vi "MeasurementControl - Main (CLTC-C0NBTZ1's conflicted copy 2015-04-20).vi"() -> ()   [LabVIEW 2013]
uses:
  Instrument Control Switches.ctl
  Timing and Stabilization/Stabilization.ctl
  avantesSpectrometer/Acquisition/Sphere Indicator.ctl
  Time Left.ctl
  controls/Metadata all typedef.ctl
  controls/Metadata typedef.ctl
  controls/Metadata disable typedef.ctl
  CaliforniaInstrumentsIxSeries/controls/electrical2.ctl
  avantesSpectrometer/Acquisition/AvaSpec Color Parameters.ctl
  MeasurementControl Message Queue Folder/MeasurementControl Message Queue.lvlib
  avantesSpectrometer/AvaSpec.lvlib
  controls/Metadata.lvlib
  CaliforniaInstrumentsIxSeries/Acquisition/Cal Inst Acquisition.lvlib
  MR 16 teardown/MR16TestStandDAQ/Controls/Stabilization.ctl
  Timing and Stabilization.lvlib
panel:
  in  "Instrument Control Switches":T1
  in  "Exit":bool
  out "Status":string
  in  "test cal inst":bool
  in  "test Yokogawa":bool
  in  "Test Naked Sphere":bool
  in  "Start LM-79\nNaked Sphere":bool
  in  "Take Measurements\nfor Database":bool
  in  "Tab Control":T2(tab)
  out "Naked Sphere Stabilization Data":T3={"Stabilization waveform"={"t0"=timestamp(0 s since 1904-01-01), "dt"=50.0, "Y"=[10.0, 9.0, 8.75, 8.5, 8.25, 8.125, 8.06, 8.03, 8.015, 8.0, 8.0, 8.0]}, "Variation"=0.0, "Stabilized"=FALSE, "Threshold"=0.0, "time to stabilize"=0.0, "3 points"=[], "Sphere Indicator"=enum."Naked Sphere"}
  out "Insulated Sphere Stabilization Data":T3={"Stabilization waveform"={"t0"=timestamp(0 s since 1904-01-01), "dt"=50.0, "Y"=[10.0, 9.0, 8.75, 8.5, 8.25, 8.125, 8.06, 8.03, 8.015, 8.0, 8.0, 8.0]}, "Variation"=0.0, "Stabilized"=FALSE, "Threshold"=0.0, "time to stabilize"=0.0, "3 points"=[], "Sphere Indicator"=enum."Naked Sphere"}
  out "Time Left":T5
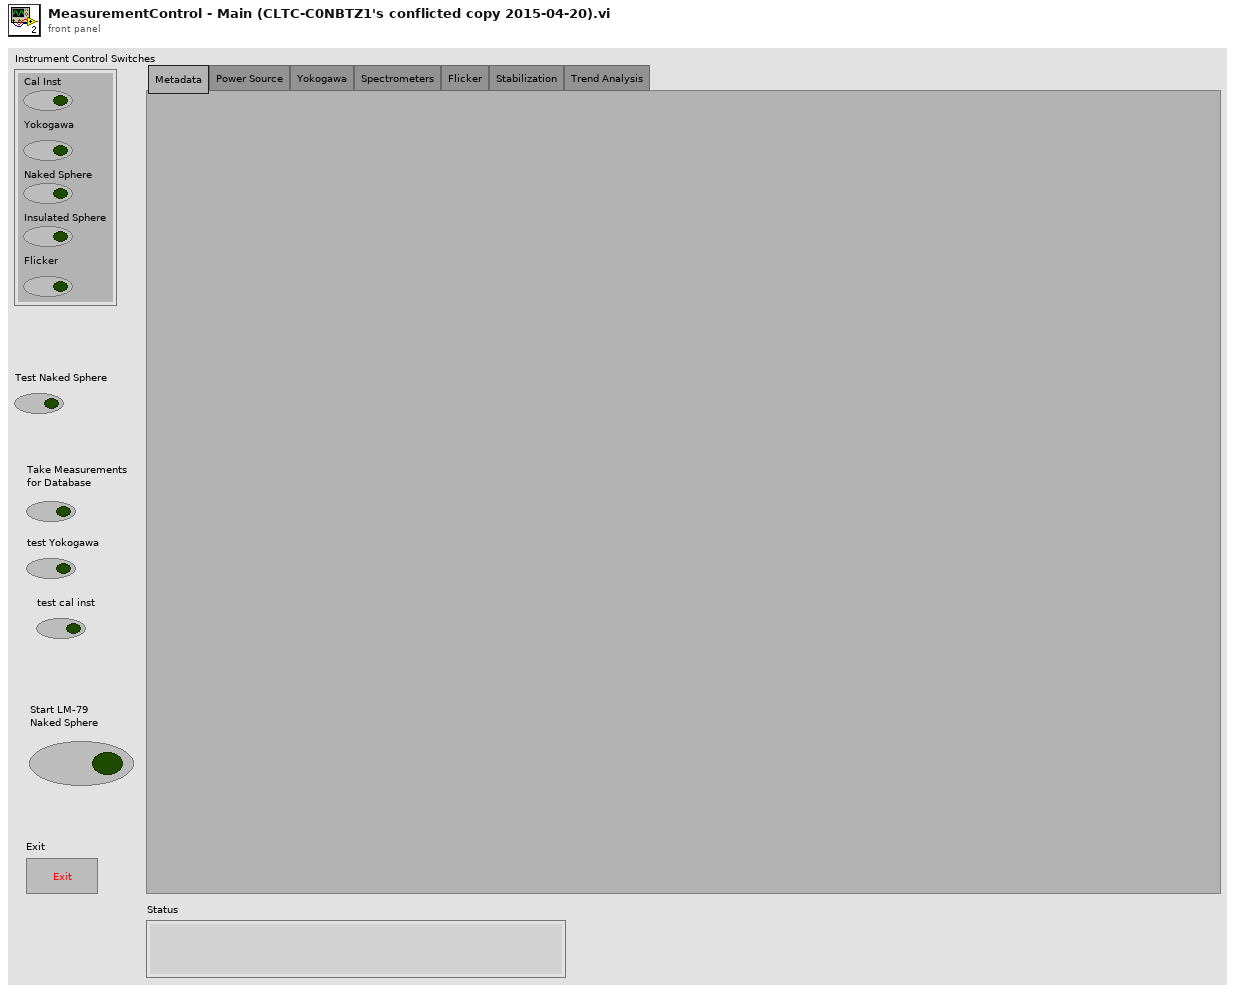
[diagram p1: front panel]
types:
  T1 = typedef "Instrument Control Switches.ctl" = cluster{"Cal Inst":bool, "Yokogawa":bool, "Naked Sphere":bool, "Insulated Sphere":bool, "Flicker":bool}
  T2 = enum32{"Metadata", "Power Source", "Yokogawa", "Spectrometers", "Flicker", "Stabilization", "Trend Analysis"}
  T3 = typedef "Timing and Stabilization.lvlib/Stabilization.ctl" = cluster{"Stabilization waveform":waveform(dbl), "Variation":dbl, "Stabilized":bool, "Threshold":dbl, "time to stabilize":dbl, "3 points":dbl[], "Sphere Indicator":T4}
  T4 = typedef "AvaSpec.lvlib/Sphere Indicator.ctl" = enum16{"Naked Sphere", "Insulated Sphere"}
  T5 = typedef "Time Left.ctl" = cluster{"Naked Sphere Time Left":dbl, "Insulated Sphere Time Left":dbl}
  T6 = typedef "Metadata.lvlib/Metadata all typedef.ctl" = cluster{"Data Fields":T7, "Metadata Disable":T8, "Output Path":path}
  T7 = typedef "Metadata.lvlib/Metadata typedef.ctl" = cluster{"operatorName":string, "project":string, "measurementType":string, "sphere":string, "spectrometer":string, "powerSource":string, "analyzer":string, "fixtureType":string, "lampType":string, "sourceType":string, "testOrientation":string, "model":string, "sample":string, "hours":string, "Amp Gain Range":string}
  T8 = typedef "Metadata.lvlib/Metadata disable typedef.ctl" = cluster{"spectrometer":enum8{"Enabled", "Disabled", "Disabled and Grayed Out"}, "sphere":enum8{"Enabled", "Disabled", "Disabled and Grayed Out"}, "analyzer":enum8{"Enabled", "Disabled", "Disabled and Grayed Out"}, "ampGainRange":enum8{"Enabled", "Disabled", "Disabled and Grayed Out"}}
  T9 = typedef "MeasurementControl Message Queue.lvlib/All Message Queues.ctl" = cluster{"Master":refnum<queue>, "UI":refnum<queue>, "Stabilization":refnum<queue>, "Logging":refnum<queue>, "Timing":refnum<queue>}
  T10 = typedef "Cal Inst.lvlib/Cal Inst Acquisition.lvlib/electrical2.ctl" = cluster{"Time Stamp":timestamp, "Temperature (C)":dbl, "Electrical Data":string[][], "Waveform Graph":waveform(dbl)[]}
  T11 = typedef "AvaSpec.lvlib/AvaSpec Color Parameters.ctl" = cluster{"Power Spectral Distribution":cluster{"X":dbl, "Y":dbl}[], "Color Values":cluster{"luminousFlux":dbl, "CCT":dbl, "CRI":dbl, "u'":dbl, "v'":dbl, "Duv":dbl}, "R values":dbl[], "Chromaticity \nCoordinates":cluster{"x":dbl, "y":dbl, "z":dbl, "u":dbl, "v":dbl}, "Tristimulus \nValues":cluster{"X":dbl, "Y":dbl, "Z":dbl}, "Time Stamp":timestamp, "Temperature":dbl, "Integration Time":dbl, "Sphere Indicator":T4}
  T12 = typedef "Stabilization.ctl" = cluster{"Stabilization waveform":waveform(dbl), "Variation":dbl, "Stabilized":bool, "Threshold":dbl, "time to stabilize":dbl, "3 points":dbl[]}
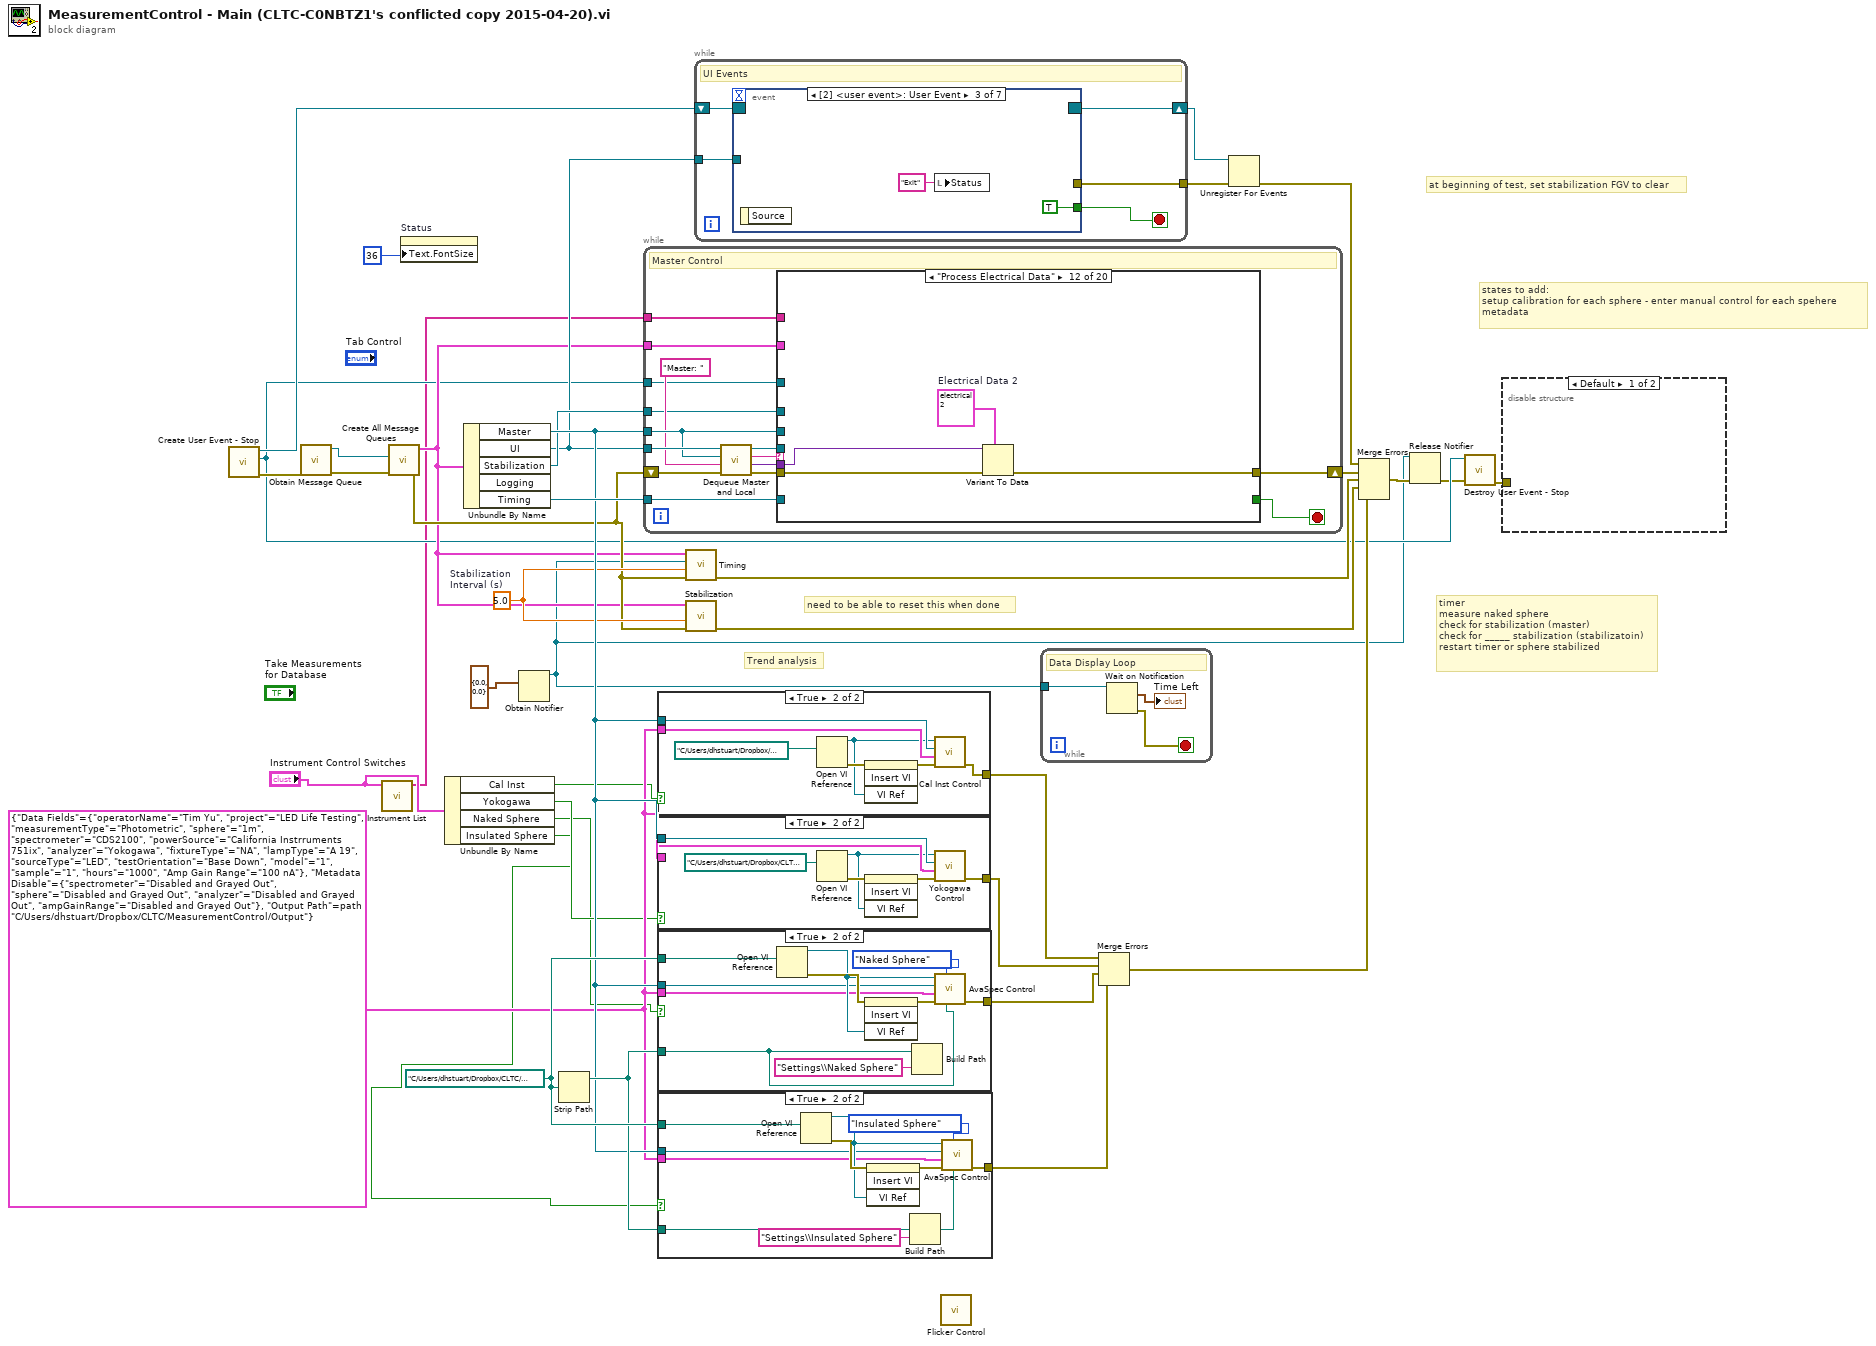
[diagram p0: block diagram]
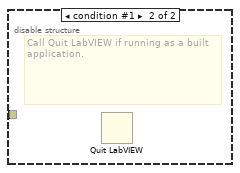
[diagram p2: hidden frame]
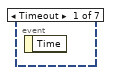
[diagram p3: hidden frame]
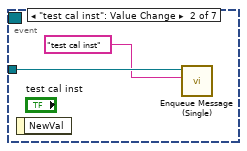
[diagram p4: hidden frame]
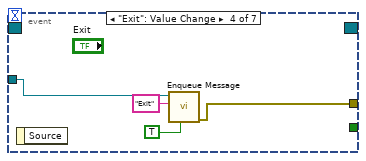
[diagram p5: hidden frame]
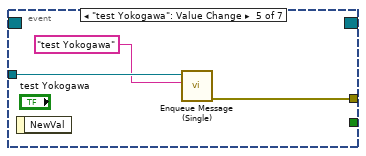
[diagram p6: hidden frame]
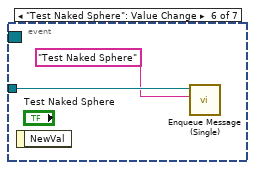
[diagram p7: hidden frame]
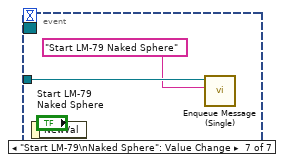
[diagram p8: hidden frame]
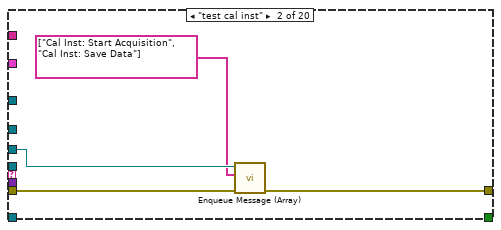
[diagram p10: hidden frame]
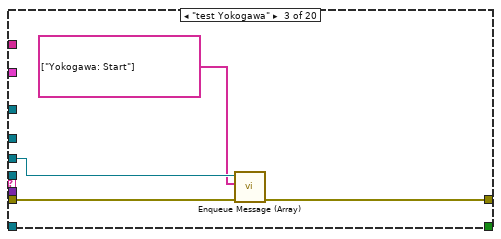
[diagram p11: hidden frame]
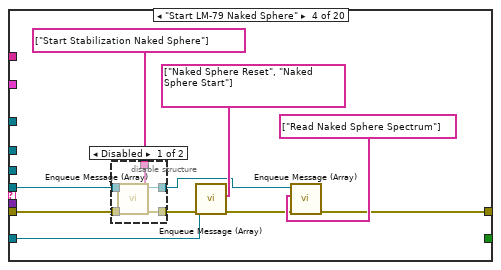
[diagram p12: hidden frame]
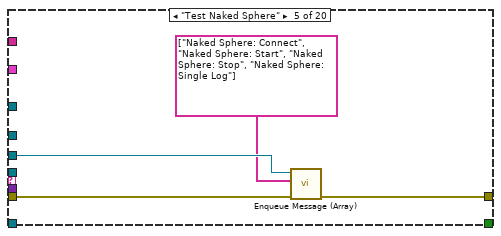
[diagram p14: hidden frame]
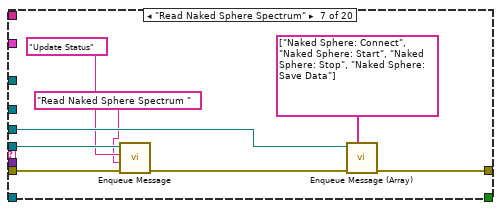
[diagram p16: hidden frame]
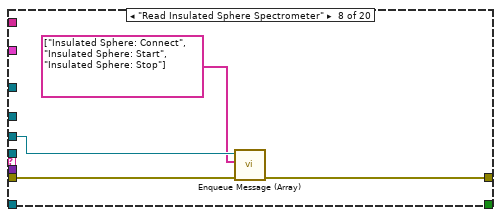
[diagram p17: hidden frame]
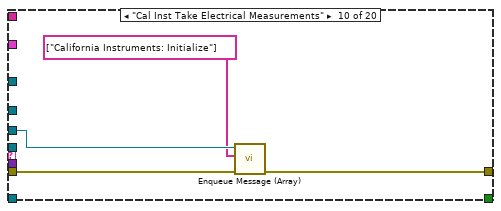
[diagram p19: hidden frame]
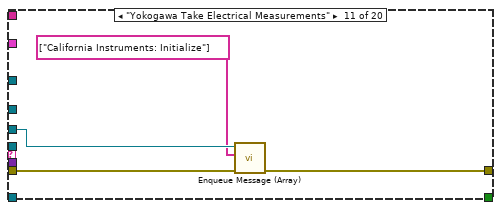
[diagram p20: hidden frame]
diagram:
  w30 = 5.0  # Stabilization Interval (s)
  w35 = path "C:/Users/dhstuart/Dropbox/CLTC/avantesSpectrometer/AvaSpec Main.vit"
  w29 = T6 {"Data Fields"={"operatorName"="Tim Yu", "project"="LED Life Testing", "measurementType"="Photometric", "sphere"="1m", "spectrometer"="CDS2100", "powerSource"="California Instrruments 751ix", "analyzer"="Yokogawa", "fixtureType"="NA", "lampType"="A 19", "sourceType"="LED", "testOrientation"="Base Down", "model"="1", "sample"="1", "hours"="1000", "Amp Gain Range"="100 nA"}, "Metadata Disable"={"spectrometer"=enum."Disabled and Grayed Out", "sphere"=enum."Disabled and Grayed Out", "analyzer"=enum."Disabled and Grayed Out", "ampGainRange"=enum."Disabled and Grayed Out"}, "Output Path"=path "C:/Users/dhstuart/Dropbox/CLTC/MeasurementControl/Output"} ("Metadata All")
  # "timer\nmeasure naked sphere\ncheck for stabilization (master)\ncheck for _____ stabilization (stabilizatoin)\nrestart timer or sphere stabilized"
  # "Trend analysis"
  # "at beginning of test, set stabilization FGV to clear"
  # "need to be able to reset this when done"
  # "states to add:\nsetup calibration for each sphere - enter manual control for each spehere\nmetadata"
  n1 = call "Create User Event - Stop.vi"() -> ("error out"=w27:errorcluster, "User Event - Stop"=w12:refnum<user-event>, "Stop Event Registration Refnum"=w23:refnum<event-registration>)  [unwired: 9 in]
  n2 = call "Obtain Message Queue.vi"("error in (no error)"=w27) -> ("error out"=w37:errorcluster, "Message Queue"=w38:refnum<queue>)  [unwired: 9 in]
  n3 = call "Instrument List.vi"("Instrument Control Switches"="Instrument Control Switches") -> ("Instrument Names"=w6:string[])  [unwired: 10 in]
  n4 = call "Create All Message Queues.vi"("error in (no error)"=w37, "Master Queue In"=w38) -> ("error out"=w28:errorcluster, "Message Queues out"=w14:T9)  [unwired: 8 in]
  n5 = property on="Status" class="Str"("Text.FontSize"=u32 36 ("Text.Font:Size")) -> ()  [unwired: 2 in, 2 out]
  n6 = Unbundle By Name("Instrument Control Switches") -> ("Cal Inst"=w11:bool, "Yokogawa"=w10:bool, "Naked Sphere"=w9:bool, "Insulated Sphere"=w8:bool)
  n7 = Unbundle By Name(w14) -> ("Master"=w33:refnum<queue>, "UI"=w31:refnum<queue>, "Stabilization"=w32:refnum<queue>, "Timing"=w36:refnum<queue>)  [unwired: 1 out]
  n8 = Obtain Notifier(notification data type=T5 {"Naked Sphere Time Left"=0.0, "Insulated Sphere Time Left"=0.0} ("Cluster 2")) -> (notifier out=w2:refnum<notifier>)  [unwired: 3 in, 2 out]
  n9 = Strip Path(path=w35) -> (stripped path=w34:path)  [unwired: 1 out]
  n10 = while {
    tunnel: w31 -> [w52]
    tunnel: w33 -> [w45]
    shift-right: [w48] -> w26
    shift-left: w28 -> [w50]
    tunnel: w36 -> [w46]
    tunnel: w32 -> [w43]
    tunnel: w14 -> [w42]
    tunnel: w12 -> [w40]
    tunnel: w6 -> [w39]
    stop <- w41 stop-if-true
    # "Master Control"
    n11 = call "Dequeue Master and Local.vi"("error in (no error)"=w50, "Instrument Name"="Master: ", "Master"=w45, "UI"=w52) -> ("error out"=w51:errorcluster, "Message Data"=w49:variant, "Message"=w53:string, "UI out"=w47:refnum<queue>)  [unwired: 4 in]
    n12 = case shown="\"Process Electrical Data\"" w53 {
      tunnel: w45 -> [_ w58 w62 _ w82 _ w91 w95 _ w100 w104 _ _ _ _ _ _ _ w159 _]
      tunnel: w51 -> [w54 w56 w60 w69 w79 w83 w88 w93 w96 w98 w102 w106 w109 w123 w128 w135 w139 w156 w171 w179]
      tunnel: w49 -> [_ _ _ _ _ _ _ _ _ _ _ w108 _ w124 w129 w136 w140 w154 _ _]
      tunnel: [w54 w55 w59 w68 w80 w83 w89 w92 w96 w97 w101 w105 w109 w121 w127 w134 w138 w155 w164 w179] -> w48
      tunnel: w47 -> [_ _ _ w71 _ _ w86 _ _ _ _ _ _ w112 _ _ _ _ w172 _]
      tunnel: w46 -> [_ _ _ w65 _ _ _ _ _ _ _ _ _ _ _ _ _ _ _ _]
      tunnel: w43 -> [_ _ _ _ _ _ _ _ _ _ _ _ _ w120 _ _ w137 _ _ _]
      tunnel: w42 -> [_ _ _ _ _ _ _ _ _ _ _ _ _ _ _ _ _ _ w173 _]
      tunnel: [_ _ _ _ _ _ _ _ _ _ _ _ _ _ _ _ _ _ TRUE _] -> w41
      tunnel: w40 -> [_ _ _ _ _ _ _ _ _ _ _ _ _ _ _ _ _ _ w166 _]
      tunnel: w39 -> [_ _ _ _ _ _ _ _ _ _ _ _ _ _ _ _ _ _ w158 _]
      frame Default {
      }
      frame "test cal inst" {
        n13 = call "Enqueue Message (Array).vi"("error in (no error)"=w56, "Message Array"=string[] ["Cal Inst: Start Acquisition", "Cal Inst: Save Data"], "Message Queue"=w58) -> ("error out"=w55:errorcluster)  [unwired: 7 in, 1 out]
      }
      frame "test Yokogawa" {
        n14 = call "Enqueue Message (Array).vi"("error in (no error)"=w60, "Message Array"=string[] ["Yokogawa: Start"], "Message Queue"=w62) -> ("error out"=w59:errorcluster)  [unwired: 7 in, 1 out]
      }
      frame "Start LM-79 Naked Sphere" {
        n15 = disable-structure shown="Disabled" {
          disable-tunnel: w71 -> [w77 w78]
          disable-tunnel: string[] ["Start Stabilization Naked Sphere"] ("Message Array") -> [w76 _]
          disable-tunnel: w69 -> [w75 _]
          disable-tunnel: [w74 _] -> w67
          disable-tunnel: [w73 w78] -> w63
          frame Disabled {
            n16 = call "Enqueue Message (Array).vi"("error in (no error)"=w75, "Message Array"=w76, "Message Queue"=w77) -> ("error out"=w74:errorcluster, "dup Message Queue"=w73:refnum<queue>)  [unwired: 7 in]
          }
          frame Enabled {
          }
        }
        n17 = call "Enqueue Message (Array).vi"("error in (no error)"=w67, "Message Array"=string[] ["Naked Sphere Reset", "Naked Sphere Start"], "Message Queue"=w65) -> ("error out"=w66:errorcluster)  [unwired: 7 in, 1 out]
        n18 = call "Enqueue Message (Array).vi"("error in (no error)"=w66, "Message Array"=string[] ["Read Naked Sphere Spectrum"], "Message Queue"=w63) -> ("error out"=w68:errorcluster)  [unwired: 7 in, 1 out]
      }
      frame "Test Naked Sphere" {
        n19 = call "Enqueue Message (Array).vi"("error in (no error)"=w79, "Message Array"=string[] ["Naked Sphere: Connect", "Naked Sphere: Start", "Naked Sphere: Stop", "Naked Sphere: Single Log"], "Message Queue"=w82) -> ("error out"=w80:errorcluster)  [unwired: 7 in, 1 out]
      }
      frame "--------Spectrometers------------" {
      }
      frame "Read Naked Sphere Spectrum" {
        n20 = call-poly "Enqueue Message.vi"("error in (no error)"=w88, "Message Data"="Read Naked Sphere Spectrum " ("Message"), "Message"="Update Status", "Message Queue"=w86) -> ("error out"=w87:errorcluster)  [unwired: 6 in, 1 out]
        n21 = call "Enqueue Message (Array).vi"("error in (no error)"=w87, "Message Array"=string[] ["Naked Sphere: Connect", "Naked Sphere: Start", "Naked Sphere: Stop", "Naked Sphere: Save Data"], "Message Queue"=w91) -> ("error out"=w89:errorcluster)  [unwired: 7 in, 1 out]
      }
      frame "Read Insulated Sphere Spectrometer" {
        n22 = call "Enqueue Message (Array).vi"("error in (no error)"=w93, "Message Array"=string[] ["Insulated Sphere: Connect", "Insulated Sphere: Start", "Insulated Sphere: Stop"], "Message Queue"=w95) -> ("error out"=w92:errorcluster)  [unwired: 7 in, 1 out]
      }
      frame "----------Electrical----------" {
      }
      frame "Cal Inst Take Electrical Measurements" {
        n23 = call "Enqueue Message (Array).vi"("error in (no error)"=w98, "Message Array"=string[] ["California Instruments: Initialize"], "Message Queue"=w100) -> ("error out"=w97:errorcluster)  [unwired: 7 in, 1 out]
      }
      frame "Yokogawa Take Electrical Measurements" {
        n24 = call "Enqueue Message (Array).vi"("error in (no error)"=w102, "Message Array"=string[] ["California Instruments: Initialize"], "Message Queue"=w104) -> ("error out"=w101:errorcluster)  [unwired: 7 in, 1 out]
      }
      frame "Process Electrical Data" {
        w107 = T10 {"Time Stamp"=timestamp(0 s since 1904-01-01), "Temperature (C)"=0.0, "Electrical Data"=[], "Waveform Graph"=[]}  # Electrical Data 2
        n25 = Variant To Data(error in=w106, type=w107, Variant=w108) -> (error out=w105:errorcluster)  [unwired: 1 out]
      }
      frame "-----------Stabilization-----------" {
      }
      frame "Check for Stabilization" {
        w118 = T11 {"Power Spectral Distribution"=[], "Color Values"={"luminousFlux"=0.0, "CCT"=0.0, "CRI"=0.0, "u'"=0.0, "v'"=0.0, "Duv"=0.0}, "R values"=[], "Chromaticity \nCoordinates"={"x"=0.0, "y"=0.0, "z"=0.0, "u"=0.0, "v"=0.0}, "Tristimulus \nValues"={"X"=0.0, "Y"=0.0, "Z"=0.0}, "Time Stamp"=timestamp(0 s since 1904-01-01), "Temperature"=0.0, "Integration Time"=0.0, "Sphere Indicator"=enum."Naked Sphere"}  # Color Parameters
        n26 = Variant To Data(error in=w123, type=w118, Variant=w124) -> (data=w119:T11, error out=w122:errorcluster)
        n27 = Unbundle By Name(w119) -> ("Sphere Indicator"=w117:T4, "Color Values.luminousFlux"=w113:dbl)
        n28 = Format Into String(w117) -> (resulting string=w116:string)  [unwired: 3 in, 1 out]
        n29 = Concatenate Strings("Check " ("Message"), w116, " Stabilization" ("Message")) -> (w110:string)
        n30 = call-poly "Enqueue Message.vi"("Message Data"=w110, "Message"="Update Status", "Message Queue"=w112) -> ()  [unwired: 7 in, 2 out]
        n31 = call-poly "Enqueue Message.vi"("error in (no error)"=w122, "Message Data"=w113, "Message"=w110, "Message Queue"=w120) -> ("error out"=w121:errorcluster)  [unwired: 6 in, 1 out]
      }
      frame "Update Stabilization" {
        n32 = Variant To Data(error in=w128, type=T3 {"Stabilization waveform"={"t0"=timestamp(0 s since 1904-01-01), "dt"=50.0, "Y"=[10.0, 9.0, 8.75, 8.5, 8.25, 8.125, 8.06, 8.03, 8.015, 8.0, 8.0, 8.0]}, "Variation"=0.0, "Stabilized"=FALSE, "Threshold"=0.0, "time to stabilize"=0.0, "3 points"=[], "Sphere Indicator"=enum."Naked Sphere"} ("Stabilization Data"), Variant=w129) -> (data=w126:T3, error out=w127:errorcluster)
        n33 = Unbundle By Name(w126) -> ("Sphere Indicator"=w125:T4)
        n34 = case shown="\"Insulated Sphere\"" w125 {
          tunnel: w126 -> [w131 w132]
          frame "Naked Sphere", Default {
            "Naked Sphere Stabilization Data" <- w131
          }
          frame "Insulated Sphere" {
            "Insulated Sphere Stabilization Data" <- w132
          }
        }
      }
      frame "Stabilization Complete" {
        # "Take other measurements"
        # "Send notification"
        # "Save Stabilization"
        n35 = Variant To Data(error in=w135, type=Sphere_Indicator."Naked Sphere" ("Sphere Indicator"), Variant=w136) -> (error out=w134:errorcluster)  [unwired: 1 out]
      }
      frame "Insulated Sphere Stabilized" {
        # "Save Stabilization Data. Save final photometric data. Collect Electrical.\nCollect flicker. Stop timer. Check trends. Send alert."
        n36 = disable-structure shown="Disabled" {
          disable-tunnel: w140 -> [w152 _]
          disable-tunnel: w139 -> [w151 _]
          disable-tunnel: [w149 _] -> w138
          disable-tunnel: w137 -> [w148 _]
          frame Disabled {
            w141 = T12 {"Stabilization waveform"={"t0"=timestamp(0 s since 1904-01-01), "dt"=1.0, "Y"=[]}, "Variation"=0.0, "Stabilized"=FALSE, "Threshold"=0.0, "time to stabilize"=0.0, "3 points"=[]}  # Stabilization Data
            n37 = Variant To Data(error in=w151, type=w141, Variant=w152) -> (data=w147:T12, error out=w150:errorcluster)
            n38 = Unbundle By Name(w147) -> ("luminousFlux"=w142)  [unwired: 1 out]
            n39 = Format Into String() -> (resulting string=w146:string)  [unwired: 4 in, 1 out]
            n40 = Concatenate Strings("Check " ("Message"), w146, " Stabilization" ("Message")) -> (w143:string)
            n41 = call-poly "Enqueue Message.vi"("error in (no error)"=w150, "Message Data"=w142, "Message"=w143, "Message Queue"=w148) -> ("error out"=w149:errorcluster)  [unwired: 6 in, 1 out]
          }
          frame Enabled {
          }
        }
      }
      frame "Update Status" {
        n42 = Variant To Data(error in=w156, type="", Variant=w154) -> (data=→"Status":string, error out=w155:errorcluster)
      }
      frame "Exit" {
        n43 = Release Queue(queue=w172, error in (no error)=w171) -> (error out=w161:errorcluster)  [unwired: 1 in, 2 out]
        n44 = call "Fire User Event - Stop.vi"("User Event - Stop"=w166) -> ("error out"=w163:errorcluster)  [unwired: 10 in]
        n45 = Cluster To Array(cluster=w173) -> (array=w169:refnum<queue>[])
        n46 = call "Exit Open Instruments.vi"("error in (no error)"=w161, "Instrument Names"=w158, "Master"=w159) -> ("error out"=w160:errorcluster)  [unwired: 8 in]
        n47 = Delete From Array(array=w169, length=2, index=0) -> (array with subset deleted=w167:refnum<queue>[])  [unwired: 1 out]
        n48 = for {
          tunnel: w167 -> [w177] mode=indexing
          shift-right: [w175] -> w165
          shift-left: w160 -> [w174]
          # "Exit all Modules"
          n49 = call "Enqueue Message (Single).vi"("error in (no error)"=w174, "Message"="Exit", "Message Queue"=w177) -> ("error out"=w175:errorcluster)  [unwired: 7 in, 1 out]
        }
        n50 = Merge Errors(w163, w165) -> (w164:errorcluster)
      }
      frame "Ignore Message" {
        n51 = Wait (ms)(milliseconds to wait=u32 500) -> ()  [unwired: 1 out]
      }
    }
  }
  n52 = case shown="True" w11 {
    tunnel: w29 -> [_ w186]
    tunnel: w33 -> [_ w185]
    tunnel: [_ w180] -> w19
    frame False {
    }
    frame True {
      n53 = Open VI Reference(vi path=path "C:/Users/dhstuart/Dropbox/CLTC/CaliforniaInstrumentsIxSeries/Cal Inst Main.vi") -> (vi reference=w181:refnum<vi>, error out=w183:errorcluster)  [unwired: 5 in]
      n54 = invoke on="California Instruments" class="SubPanel" method="Insert VI"(error in=w183, "VI Ref"=w181) -> (error out=w182:errorcluster)  [unwired: 2 in, 3 out]
      n55 = call "Cal Inst Control.vi"("error in (no error)"=w182, "Metadata All"=w186, "Master"=w185, "VI in"=w181) -> ("error out"=w180:errorcluster)  [unwired: 6 in, 1 out]
    }
  }
  n56 = case shown="True" w10 {
    tunnel: w33 -> [_ w190]
    tunnel: w29 -> [_ w191]
    tunnel: [_ w187] -> w18
    frame False {
    }
    frame True {
      n57 = Open VI Reference(vi path=path "C:/Users/dhstuart/Dropbox/CLTC/YokogawaPZ4000/YKPZ400 main.vi") -> (vi reference=w189:refnum<vi>, error out=w192:errorcluster)  [unwired: 5 in]
      n58 = invoke on="Yokogawa" class="SubPanel" method="Insert VI"(error in=w192, "VI Ref"=w189) -> (error out=w188:errorcluster)  [unwired: 2 in, 3 out]
      n59 = call "Yokogawa Control.vi"("error in (no error)"=w188, "Metadata All"=w191, "Master"=w190, "VI in"=w189) -> ("error out"=w187:errorcluster)  [unwired: 6 in, 1 out]
    }
  }
  n60 = case shown="True" w9 {
    tunnel: w35 -> [_ w200]
    tunnel: w34 -> [_ w194]
    tunnel: w33 -> [_ w197]
    tunnel: w29 -> [_ w196]
    tunnel: [_ w195] -> w17
    frame False {
    }
    frame True {
      n61 = Open VI Reference(vi path=w200) -> (vi reference=w202:refnum<vi>, error out=w203:errorcluster)  [unwired: 5 in]
      n62 = invoke on="Naked Sphere" class="SubPanel" method="Insert VI"(error in=w203, "VI Ref"=w202) -> (error out=w201:errorcluster)  [unwired: 2 in, 3 out]
      n63 = Build Path(base path=w194, name or relative path="Settings\\Naked Sphere") -> ()  [unwired: 1 out]
      n64 = call "AvaSpec Control.vi"("Path"=w194, "Sphere Indicator"=Sphere_Indicator."Naked Sphere", "error in (no error)"=w201, "Metadata All"=w196, "Master"=w197, "VI in"=w202) -> ("error out"=w195:errorcluster)  [unwired: 4 in, 1 out]
    }
  }
  n65 = case shown="True" w8 {
    tunnel: w35 -> [_ w214]
    tunnel: w34 -> [_ w210]
    tunnel: w33 -> [_ w206]
    tunnel: w29 -> [_ w205]
    tunnel: [_ w204] -> w16
    frame False {
    }
    frame True {
      n66 = Open VI Reference(vi path=w214) -> (vi reference=w211:refnum<vi>, error out=w213:errorcluster)  [unwired: 5 in]
      n67 = invoke on="Insulated Sphere" class="SubPanel" method="Insert VI"(error in=w213, "VI Ref"=w211) -> (error out=w212:errorcluster)  [unwired: 2 in, 3 out]
      n68 = Build Path(base path=w210, name or relative path="Settings\\Insulated Sphere") -> (appended path=w208:path)
      n69 = call "AvaSpec Control.vi"("Path"=w208, "Sphere Indicator"=Sphere_Indicator."Insulated Sphere", "error in (no error)"=w212, "Metadata All"=w205, "Master"=w206, "VI in"=w211) -> ("error out"=w204:errorcluster)  [unwired: 4 in, 1 out]
    }
  }
  n70 = call "Timing.vi"("error in"=w28, "Stabilization\nInterval (s)"=w30, "Time Left"=w2, "Message Queues out"=w14) -> ("error out"=w21:errorcluster)  [unwired: 7 in]
  n71 = call "Stabilization.vi"("error in (no error)"=w28, "Stabilization\nInterval"=w30, "Message Queues out"=w14) -> ("error out"=w20:errorcluster)  [unwired: 8 in]
  n72 = while {
    tunnel: w31 -> [w219]
    shift-right: [w218] -> w24
    shift-left: w23 -> [w217]
    tunnel: [w215] -> w22
    stop <- w216 stop-if-true
    # "UI Events"
    n73 = event shown="[2] <user event>: User Event" {
      selector: w217 -> [_ _ _ _ _ _ _]
      dyn-events: [_ _ _ _ _ _ _] -> w218
      timeout: _ -> [_ _ _ _ _ _ _]
      tunnel: w219 -> [_ w221 _ w227 w230 w232 w234]
      tunnel: [_ _ TRUE _ _ _ _] -> w216
      tunnel: [_ _ _ w225 w228 _ _] -> w215
      event Timeout {
        n74 = event-data() -> ()  [unwired: 1 in, 1 out]
      }
      event "test cal inst": Value Change {
        n75 = event-data() -> ()  [unwired: 1 in, 1 out]
        n76 = call "Enqueue Message (Single).vi"("Message"="test cal inst", "Message Queue"=w221) -> ()  [unwired: 8 in, 2 out]
      }
      event User Event {
        n77 = event-data() -> ()  [unwired: 1 in, 1 out]
        n78 = local write "Status"("Exit" ("Status")) -> ()
      }
      event "Exit": Value Change {
        n79 = event-data() -> ()  [unwired: 1 in, 1 out]
        n80 = call-poly "Enqueue Message.vi"("Priority Message? (F)"=TRUE, "Message"="Exit", "Message Queue"=w227) -> ("error out"=w225:errorcluster)  [unwired: 7 in, 1 out]
      }
      event "test Yokogawa": Value Change {
        n81 = event-data() -> ()  [unwired: 1 in, 1 out]
        n82 = call "Enqueue Message (Single).vi"("Message"="test Yokogawa", "Message Queue"=w230) -> ("error out"=w228:errorcluster)  [unwired: 8 in, 1 out]
      }
      event "Test Naked Sphere": Value Change {
        n83 = event-data() -> ()  [unwired: 1 in, 1 out]
        n84 = call "Enqueue Message (Single).vi"("Message"="Test Naked Sphere", "Message Queue"=w232) -> ()  [unwired: 8 in, 2 out]
      }
      event "Start LM-79\nNaked Sphere": Value Change {
        n85 = event-data() -> ()  [unwired: 1 in, 1 out]
        n86 = call "Enqueue Message (Single).vi"("Message"="Start LM-79 Naked Sphere", "Message Queue"=w234) -> ()  [unwired: 8 in, 2 out]
      }
    }
  }
  n87 = call "Flicker Control.vi"() -> ()  [unwired: 12 in]
  n88 = while {
    tunnel: w2 -> [w235]
    stop <- w237 stop-if-true
    # "Data Display Loop"
    n89 = Wait on Notification(notifier=w235) -> (notification=→"Time Left":T5, error out=w237:errorcluster)  [unwired: 3 in, 2 out]
  }
  n90 = Merge Errors(w19, w18, w17, w16) -> (w15:errorcluster)
  n91 = Unregister For Events(event registration refnum=w24, error in=w22) -> (error out=w25:errorcluster)
  n92 = Merge Errors(w25, w26, w21, w20, w15) -> (w4:errorcluster)
  n93 = Release Notifier(notifier=w2, error in (no error)=w4) -> (error out=w3:errorcluster)  [unwired: 1 in, 2 out]
  n94 = call "Destroy User Event - Stop.vi"("error in (no error)"=w3, "User Event - Stop"=w12) -> ("error out"=w13:errorcluster)  [unwired: 9 in]
  n95 = disable-structure shown="Default" {
    disable-tunnel: w13 -> [_ _]
    frame condition #0 (active) {
    }
    frame condition #1 {
      # "Call Quit LabVIEW if running as a built application."
      n96 = Quit LabVIEW() -> ()  [unwired: 1 in]
    }
  }
